vi "unpackAutonArray.vi"(0 "all rows":dbl[][](array[numeric])) -> (17 "Misc 6":dbl[](array[numeric]), 19 "Misc 5":dbl[](array[numeric]), 20 "Primitive":i16[](array[numeric]), 21 "Desired Heading":dbl[](array[numeric]), 22 "Time/Distance":dbl[](array[numeric]), 23 "Power":dbl[](array[numeric]), 24 "Ramp Actuator":dbl[](array[numeric]), 25 "Harvester":dbl[](array[numeric]), 26 "Conveyor":dbl[](array[numeric]), 27 "Shoot":dbl[](array[numeric]))   [LabVIEW 2011]
doc: "Use this VI to separate the autonomous array data into individual arrays. First array is Primitive ID, second is heading, etc."
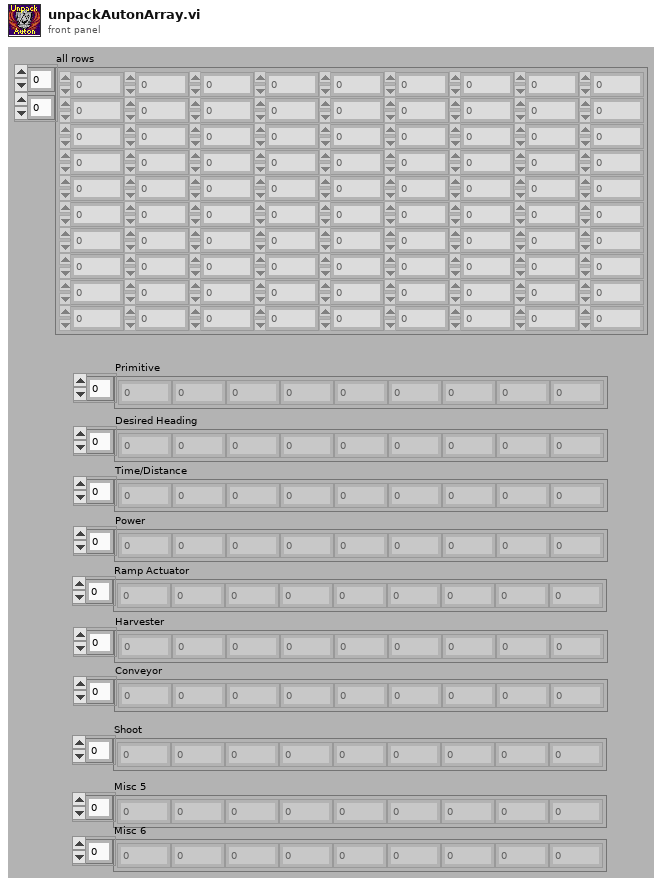
[diagram p1: front panel]
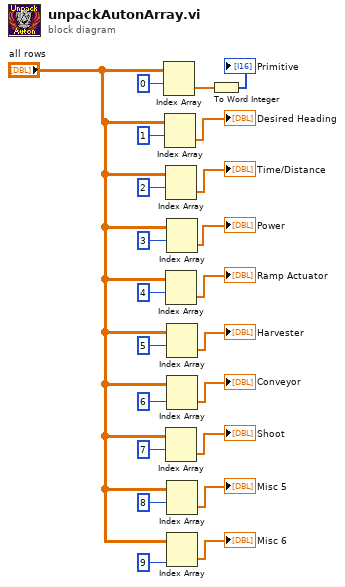
[diagram p0: block diagram]
diagram:
  n1 = Index Array(array="all rows", index (row)=0) -> (element=w19:dbl[])  [unwired: 1 in]
  n2 = Index Array(array="all rows", index (row)=1) -> (element=→"Desired Heading":dbl[])  [unwired: 1 in]
  n3 = Index Array(array="all rows", index (row)=2) -> (element=→"Time/Distance":dbl[])  [unwired: 1 in]
  n4 = Index Array(array="all rows", index (row)=4) -> (element=→"Ramp Actuator":dbl[])  [unwired: 1 in]
  n5 = Index Array(array="all rows", index (row)=7) -> (element=→"Shoot":dbl[])  [unwired: 1 in]
  n6 = Index Array(array="all rows", index (row)=3) -> (element=→"Power":dbl[])  [unwired: 1 in]
  n7 = Index Array(array="all rows", index (row)=5) -> (element=→"Harvester":dbl[])  [unwired: 1 in]
  n8 = Index Array(array="all rows", index (row)=6) -> (element=→"Conveyor":dbl[])  [unwired: 1 in]
  n9 = Index Array(array="all rows", index (row)=8) -> (element=→"Misc 5":dbl[])  [unwired: 1 in]
  n10 = Index Array(array="all rows", index (row)=9) -> (element=→"Misc 6":dbl[])  [unwired: 1 in]
  n11 = To Word Integer(number=w19) -> (16bit integer=→"Primitive":i16[])
